vi "newElf.vi"(8 "error in (no error)":errorcluster, 10 "Index":i32) -> (0 "error out":errorcluster, 3 "Elf out":refnum<class "Elf.lvclass">)   [LabVIEW 2017, in "Elf.lvclass"]
uses:
  Elf.lvclass
  Elf.lvclass/Elf.ctl
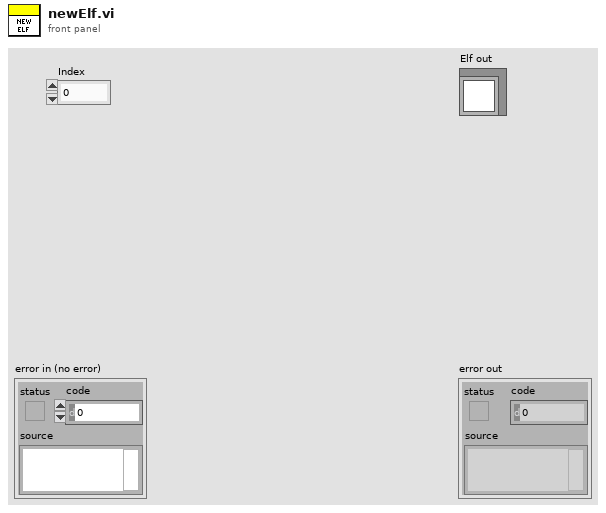
[diagram p1: front panel]
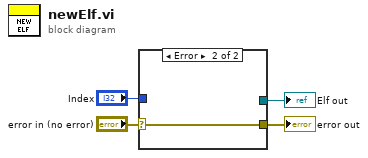
[diagram p0: block diagram]
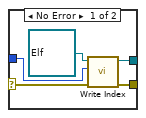
[diagram p2: hidden frame]
diagram:
  n1 = case shown="Error" "error in (no error)" {
    selector: "error in (no error)" -> [w6 w10]
    tunnel: [w5 w10] -> w3
    tunnel: [w8 _] -> w2
    tunnel: "Index" -> [w7 _]
    frame No Error {
      n2 = call "Write Index.vi"("error in (no error)"=w6, "Index"=w7, "Elf in"=refnum<class "Elf.lvclass"> refnum ("Elf.lvclass")) -> ("error out"=w5:errorcluster, "Elf out"=w8:refnum<class "Elf.lvclass">)  [unwired: 7 in]
    }
    frame Error {
    }
  }
  "error out" <- w3
  "Elf out" <- w2
